vi "Get 1D Array String.vi"(5 "use temporary file? (F)":bool, 7 "data type of variable":string[](array[string]), 8 "error in":errorcluster, 10 "variable name":string, 11 "GOLPI ref. in":T1={"pipe handle"={"lv_proc.dll file path"=path "", "process instance handle"=[], "debug mode"=FALSE, "debug data"=[]}, "fast read timeout [ms]"=500, "fast read settle time [ms]"=10, "fast read to multiple [ms]"=1, "max elements per input line"=100, "slow read timeout [ms]"=5000, "stdin double format specifier"="%_16e", "max elements per stdout output column"=100, "console mode bitstream"=FALSE, "bitstream first read timeout [ms]"=1000, "bitstream read timeout [ms]"=50, "struct transfer possible"=FALSE, "matlab mode"=FALSE, "var pipe write timeout [ms]"=5000, "variable pipe mode"=FALSE, "variable pipe buffer size [Bytes]"=10000000, "variable pipe block size [Bytes]"=1000000} {"variable pipe block size [Bytes]" format="%.0p"; "variable pipe buffer size [Bytes]" format="%.0p"}) -> (0 "error out":errorcluster, 2 "value":string[](array[string]), 3 "GOLPI ref. out":T1={"pipe handle"={"lv_proc.dll file path"=path "", "process instance handle"=[], "debug mode"=FALSE, "debug data"=[]}, "fast read timeout [ms]"=500, "fast read settle time [ms]"=10, "fast read to multiple [ms]"=1, "max elements per input line"=100, "slow read timeout [ms]"=5000, "stdin double format specifier"="%_16e", "max elements per stdout output column"=100, "console mode bitstream"=FALSE, "bitstream first read timeout [ms]"=1000, "bitstream read timeout [ms]"=50, "struct transfer possible"=FALSE, "matlab mode"=FALSE, "var pipe write timeout [ms]"=5000, "variable pipe mode"=FALSE, "variable pipe buffer size [Bytes]"=10000000, "variable pipe block size [Bytes]"=1000000} {"variable pipe block size [Bytes]" format="%.0p"; "variable pipe buffer size [Bytes]" format="%.0p"})   [LabVIEW 2020, in "GOLPI library.lvlib"]
doc: "Part of polymorph Get Variable.vi"
uses:
  GOLPI library.lvlib
  Public/GOLPI reference Type Def.ctl
  LV Process source distribution/Pipe Handle.ctl
  Type Definitions/Bitstream Data Type.ctl
  Type Definitions/Custom Error Codes Enum Type Def.vi
  LV Process source distribution/LV Process library.lvlib
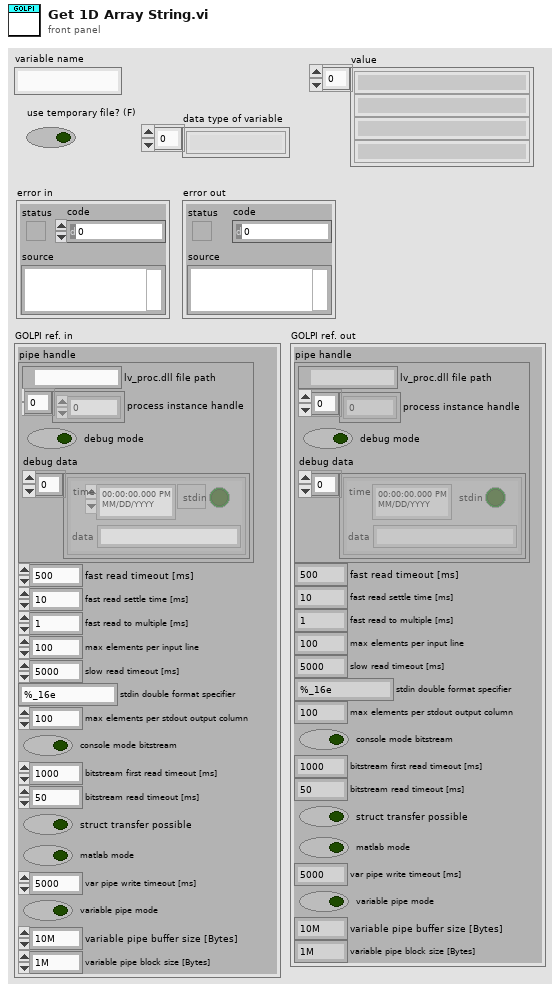
[diagram p1: front panel]
types:
  T1 = typedef "GOLPI library.lvlib/GOLPI reference Type Def.ctl" = cluster{"pipe handle":T2, "fast read timeout [ms]":u32, "fast read settle time [ms]":u32, "fast read to multiple [ms]":u32, "max elements per input line":u32, "slow read timeout [ms]":u32, "stdin double format specifier":string, "max elements per stdout output column":u32, "console mode bitstream":bool, "bitstream first read timeout [ms]":u32, "bitstream read timeout [ms]":u32, "struct transfer possible":bool, "matlab mode":bool, "var pipe write timeout [ms]":u32, "variable pipe mode":bool, "variable pipe buffer size [Bytes]":u32, "variable pipe block size [Bytes]":u32}
  T2 = typedef "LV Process library.lvlib/Pipe Handle.ctl" = cluster{"lv_proc.dll file path":path, "process instance handle":u32[], "debug mode":bool, "debug data":cluster{"time":timestamp, "stdin":bool, "data":string}[]}
  T3 = typedef "GOLPI library.lvlib/Custom Error Codes Enum Type Def.vi" = enum16{"no error", "00 working directory PAR1 missing", "01 octave binary PAR1 missing", "02 octave report error PAR1", "03 empty output last cmd PAR1", "04 missing temporary file PAR1", "05 pwd PAR 1 not exist", "06 oct package not installed", "07 octave default binary missing", "10 var PAR1 not string, vect", "11 var PAR1 not num, scal, ~compl", "12 var PAR1 not num, scal, compl", "13 var PAR1 not num, vect, ~compl", "14 var PAR1 not num, vect, compl", "15 var PAR1 not num, mat, ~compl", "16 var PAR1 not num, mat, ~compl", "30 read timeout", "60 bitstream transport failed", "61 bitstream decode error PAR1", "62 bitstream cannot be set", "70 struct transfer not possible", "80 struct: cluster elem. PAR1 not implem.", "81 struct: structure field PAR1 not implem.", "82 struct: size mismatch of PAR1", "83 struct: type mismatch of PAR1", "98 internal error", "99 not finished", "90 Not supported in Matlab mode", "91 Matlab variable transfer error", "92 Matlab Script Error"}
  T4 = typedef "GOLPI library.lvlib/Bitstream Data Type.ctl" = enum16{"dummy", "int", "uint", "float", "complex", "str", "real numeric"}
  T5 = typedef "GOLPI library.lvlib/Transfer Mode.ctl" = enum16{"Matlab", "stdio", "temp file", "bitstream", "pipe"}
  T6 = typedef "GOLPI library.lvlib/Bitstream Data.ctl" = cluster{"double":dbl[][], "cplx double":cdb[][], "int64":i64[][], "uint64":u64[][], "str":string[], "data type":T4}
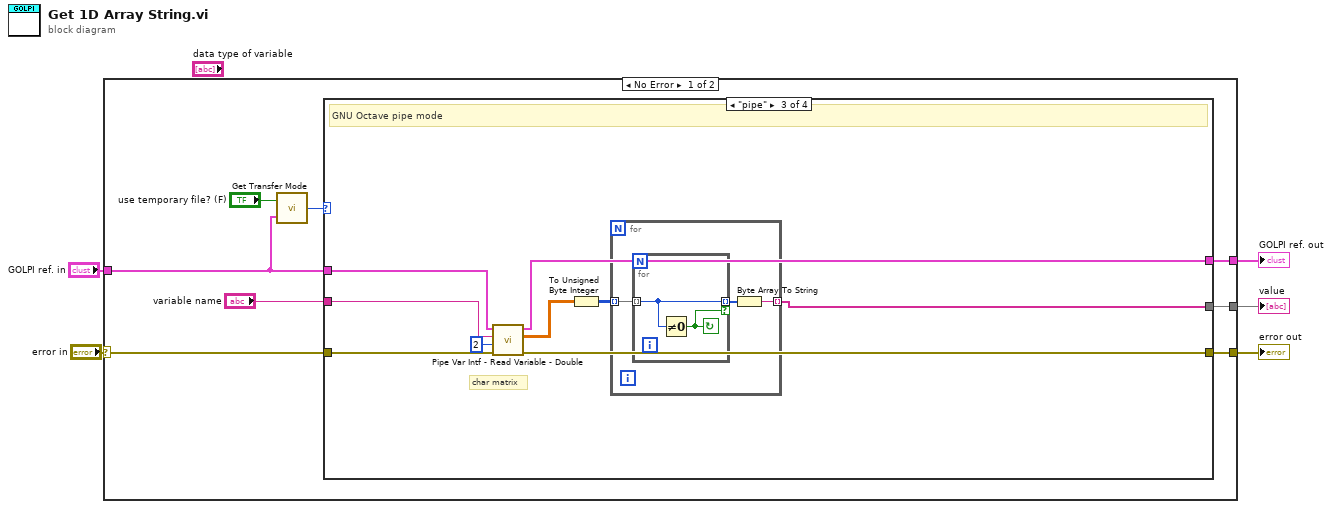
[diagram p0: block diagram]
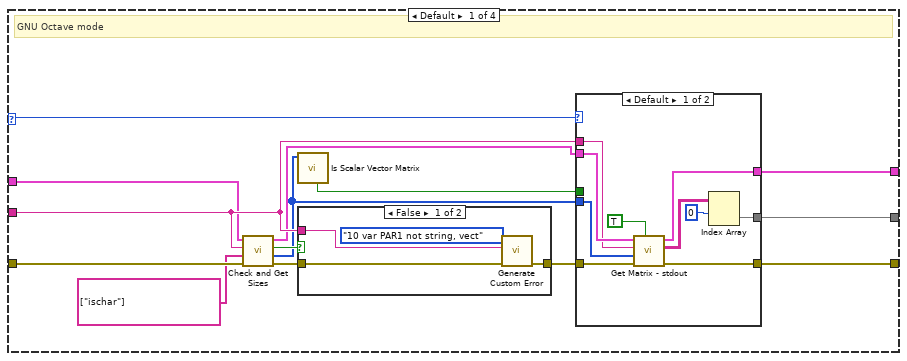
[diagram p2: hidden frame]
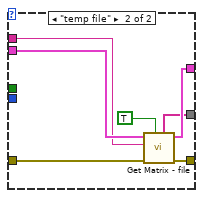
[diagram p3: hidden frame]
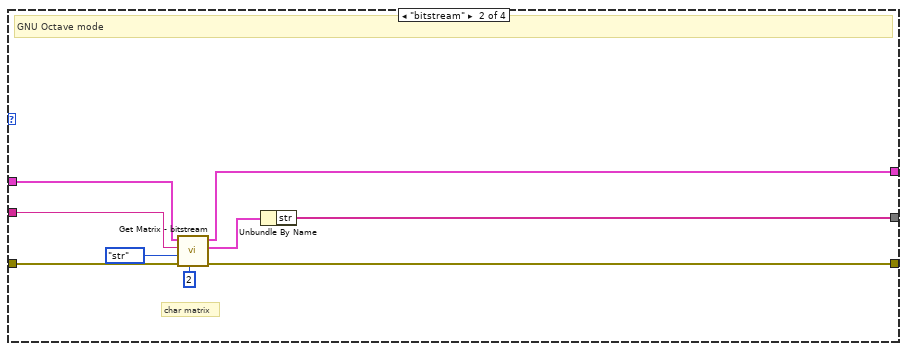
[diagram p5: hidden frame]
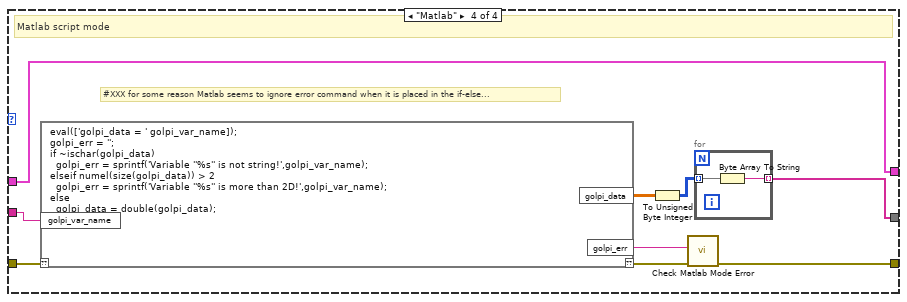
[diagram p6: hidden frame]
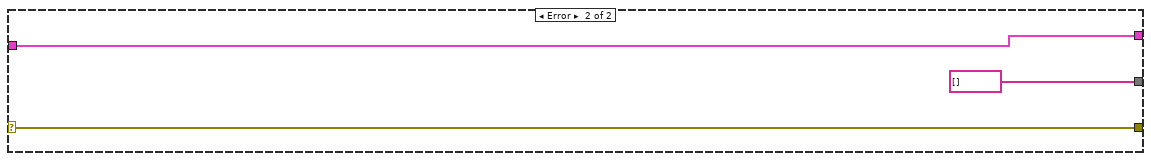
[diagram p7: hidden frame]
diagram:
  n1 = case shown="No Error" "error in" {
    selector: "error in" -> [w12 w86]
    tunnel: [w11 w86] -> w5
    tunnel: [w13 string[] [] ("vector")] -> w3
    tunnel: "GOLPI ref. in" -> [w8 w84]
    tunnel: [w9 w84] -> w1
    frame No Error {
      n2 = call "Get Transfer Mode.vi"("GOLPI ref."=w8, "use temporary file? (F)"="use temporary file? (F)") -> ("mode"=w7:T5)
      n3 = case shown="\"pipe\"" w7 {
        selector: w7 -> [w14 _ _ _]
        tunnel: [w27 w58 w59 w76] -> w13
        tunnel: w12 -> [w26 w57 w67 w81]
        tunnel: [w25 w56 w66 w73] -> w11
        tunnel: "variable name" -> [w24 w55 w65 w80]
        tunnel: [w23 w54 w64 w79] -> w9
        tunnel: w8 -> [w22 w53 w63 w79]
        frame Default {
          # "GNU Octave mode"
          n4 = call "Check and Get Sizes.vi"("error in (no error)"=w26, "test commands"=string[] ["ischar"], "variable name"=w24, "GOLPI ref. in"=w22) -> ("error out"=w20:errorcluster, "octave sizes"=w16:i32[], "all tests OK?"=w21:bool, "GOLPI ref. out"=w18:T1)  [unwired: 4 in]
          n5 = call "Is Scalar Vector Matrix.vi"("octave sizes"=w16) -> ("row vector?"=w15:bool)  [unwired: 5 in, 5 out]
          n6 = case shown="False" w21 {
            tunnel: w20 -> [w48 w49]
            tunnel: [w45 w49] -> w17
            tunnel: w24 -> [w46 _]
            frame False {
              n7 = call "Generate Custom Error.vi"("error in"=w48, "PAR1"=w46, "GOLPI error"=Custom_Error_Codes_Enum_Type_Def.vi."10 var PAR1 not string, vect" ("Enum")) -> ("error out"=w45:errorcluster)  [unwired: 8 in]
            }
            frame True {
            }
          }
          n8 = case shown="Default" w14 {
            tunnel: [w28 w39] -> w27
            tunnel: w18 -> [w37 w42]
            tunnel: w16 -> [w30 _]
            tunnel: w17 -> [w36 w44]
            tunnel: [w35 w43] -> w25
            tunnel: w24 -> [w29 w40]
            tunnel: [w34 w41] -> w23
            tunnel: w15 -> [_ _]
            frame Default {
              n9 = call "Get Matrix - stdout.vi"("is string?"=TRUE ("is string"), "error in (no error)"=w36, "octave sizes"=w30, "variable name"=w29, "GOLPI ref. in"=w37) -> ("error out"=w35:errorcluster, "array"=w31:string[][], "GOLPI ref. out"=w34:T1)  [unwired: 4 in]
              n10 = Index Array(array=w31, index (row)=0) -> (element=w28:string[])  [unwired: 1 in]
            }
            frame "temp file" {
              n11 = call "Get Matrix - file.vi"("is string?"=TRUE ("is string"), "error in (no error)"=w44, "variable name"=w40, "GOLPI ref. in"=w42) -> ("error out"=w43:errorcluster, "GOLPI ref. out"=w41:T1, "string array"=w39:string[])  [unwired: 3 in, 2 out]
            }
          }
        }
        frame "bitstream" {
          # "char matrix"
          # "GNU Octave mode"
          n12 = call "Get Matrix - bitstream.vi"("max dimensions (0: scalar)"=2, "error in (no error)"=w57, "data type"=Bitstream_Data_Type."str", "variable name"=w55, "GOLPI ref. in"=w53) -> ("error out"=w56:errorcluster, "data"=w50:T6, "GOLPI ref. out"=w54:T1)  [unwired: 4 in]
          n13 = Unbundle By Name(w50) -> ("str"=w58:string[])
        }
        frame "pipe" {
          # "char matrix"
          # "GNU Octave pipe mode"
          n14 = call "Pipe Var Intf - Read Variable - Double.vi"("error in (no error)"=w67, "max dims (0: scalar)"=2 ("max dimensions (0: scalar)"), "variable name"=w65, "GOLPI ref. in"=w63) -> ("error out"=w66:errorcluster, "data out"=w61:dbl[][], "GOLPI ref. out"=w64:T1)  [unwired: 5 in]
          n15 = To Unsigned Byte Integer(number=w61) -> (unsigned 8bit integer=w60:u8[][])
          n16 = for {
            tunnel: w60 -> [w70] mode=indexing
            tunnel: [w68] -> w59 mode=indexing
            n17 = for {
              tunnel: w70 -> [w72] mode=indexing
              tunnel: [w72] -> w69 mode=indexing if=w71
              stop <- w71 continue-if-true
              n18 = Not Equal To 0?(x=w72) -> (x != 0?=w71:bool)
            }
            n19 = Byte Array To String(unsigned byte array=w69) -> (string=w68:string)
          }
        }
        frame "Matlab" {
          # "#XXX for some reason Matlab seems to ignore error command when it is placed in the if-else..."
          # "Matlab script mode"
          n20 = script code="eval(['golpi_data = ' golpi_var_name]);\ngolpi_err = '';\nif ~ischar(golpi_data)\n  golpi_err = sprintf('Variable ''%s'' is not string!',golpi_var_name);  \nelseif numel(size(golpi_data)) > 2\n  golpi_err = sprintf('Variable ''%s'' is more than 2D!',golpi_var_name);  \nelse\n  golpi_data = double(golpi_data);\nend"("??"=w81, "golpi_var_name"=w80) -> ("??"=w75:errorcluster, "golpi_data"=w78:dbl[][], "golpi_err"=w74:string)
          n21 = To Unsigned Byte Integer(number=w78) -> (unsigned 8bit integer=w77:u8[][])
          n22 = call "Check Matlab Mode Error.vi"("error in"=w75, "custom error string (empty)"=w74) -> ("error out"=w73:errorcluster)  [unwired: 9 in]
          n23 = for {
            tunnel: w77 -> [w83] mode=indexing
            tunnel: [w82] -> w76 mode=indexing
            n24 = Byte Array To String(unsigned byte array=w83) -> (string=w82:string)
          }
        }
      }
    }
    frame Error {
    }
  }
  "value" <- w3
  "error out" <- w5
  "GOLPI ref. out" <- w1
